vi "Sensors - Create New Calibration Table from File.vi"(0 "Calibration Data File":path, 5 "Conversion Type":T1, 9 "New Calibration Data File":path, 11 "Write table to file":bool) -> (4 "Output Table":dbl[][](array[numeric]) format="%.4f")   [LabVIEW 2011]
uses:
  Sensors - Controls/Sensors - Conversion Type.ctl
  <vilib>/Analysis/NI_AALPro.lvlib
panel:
  out "Table - Original & Created Data":cluster{dbl[], dbl[]}[](graph)
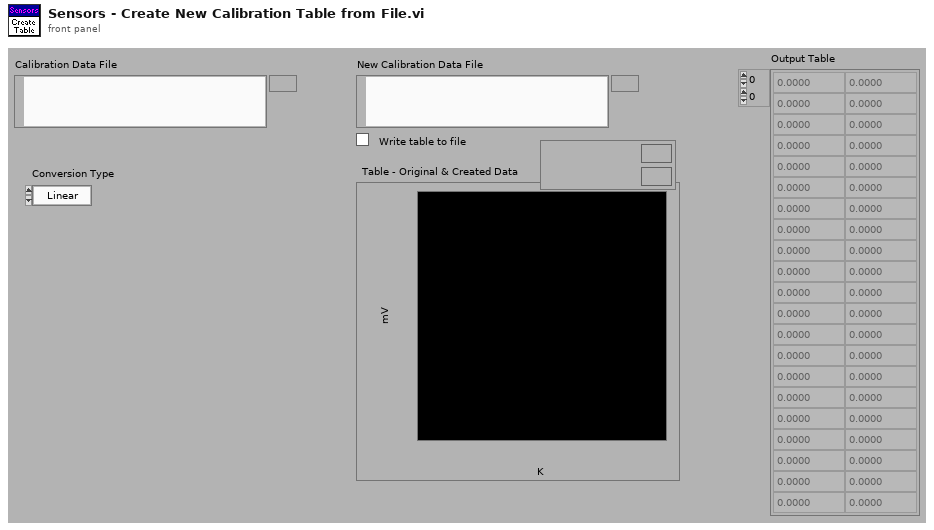
[diagram p1: front panel]
types:
  T1 = typedef "Sensors - Conversion Type.ctl" = enum16{"Linear", "Spline"}
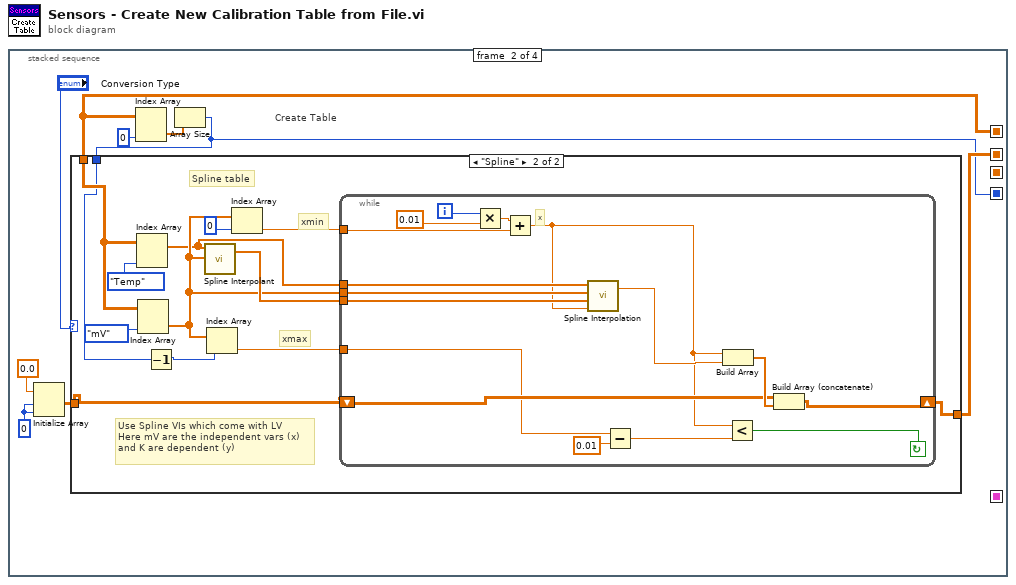
[diagram p0: block diagram]
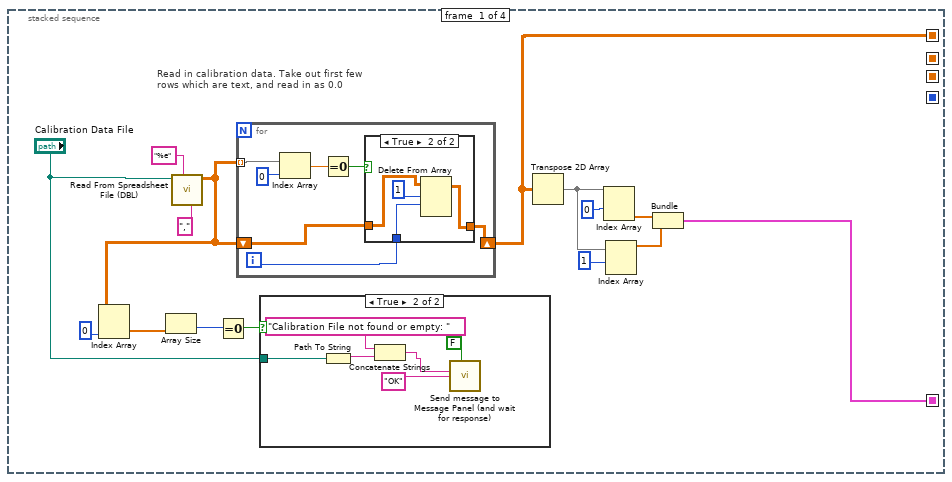
[diagram p2: hidden frame]
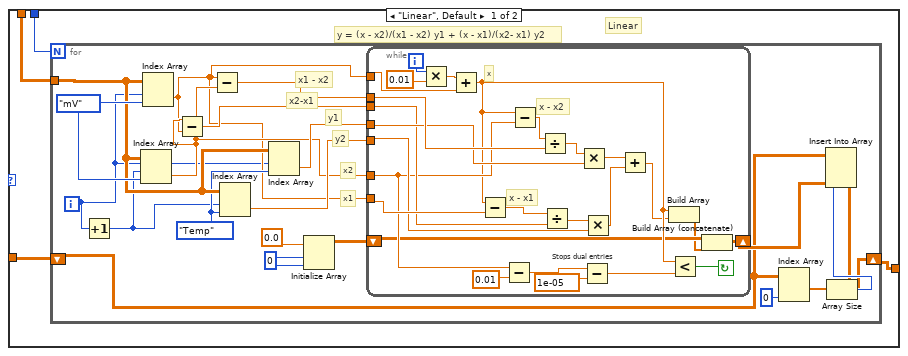
[diagram p5: hidden frame]
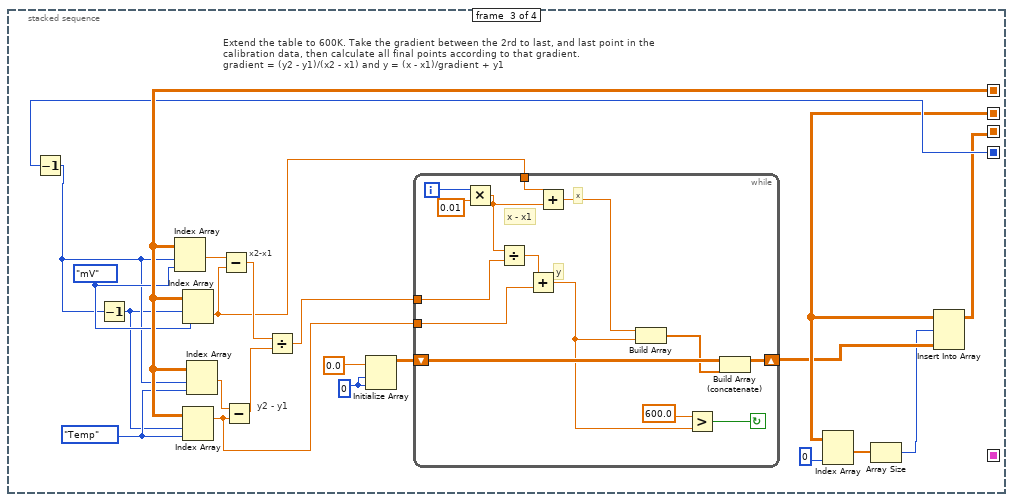
[diagram p6: hidden frame]
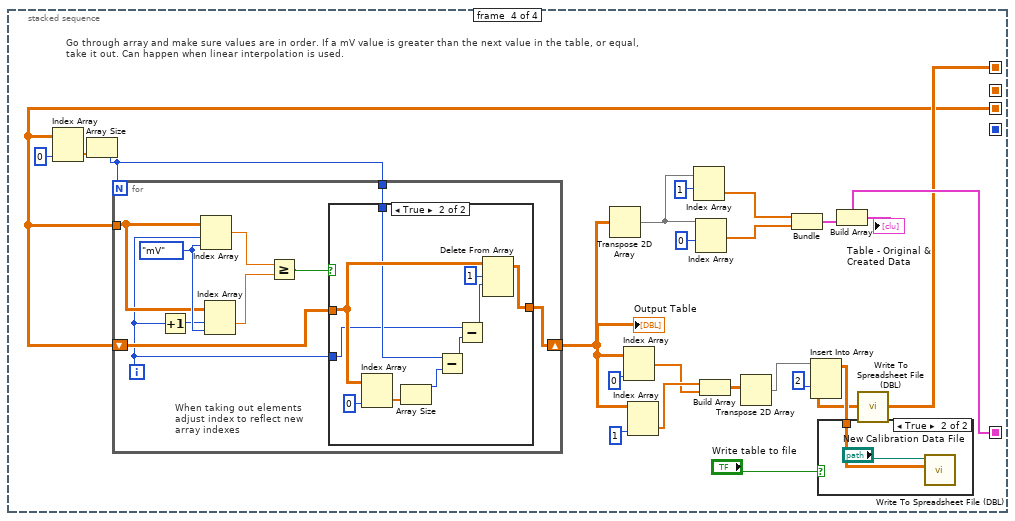
[diagram p7: hidden frame]
diagram:
  n1 = stacked-sequence {
    seq-local: [w8 _ _ _] -> [_ w37 w143 w163]
    seq-local: [_ w36 _ _] -> [_ _ w141 _]
    seq-local: [w1 _ _ _] -> [_ _ _ w172]
    seq-local: [_ w35 _ _] -> [_ _ w142 _]
    seq-local: [_ _ w140 _] -> [_ _ _ w161]
    frame #0 {
      # "Read in calibration data. Take out first few\nrows which are text, and read in as 0.0"
      n2 = call <vilib>:"Read From Spreadsheet File (DBL).vi"("delimiter (\\t)"=",", "format (%.3f)"="%e", "file path (dialog if empty)"="Calibration Data File") -> ("all rows"=w6:dbl[][])  [unwired: 4 in, 4 out]
      n3 = Index Array(array=w6, index (col)=0) -> (element=w4:dbl[])  [unwired: 1 in]
      n4 = Array Size(array=w4) -> (size(s)=w7:i32)
      n5 = Equal To 0?(x=w7) -> (x = 0?=w3:bool)
      n6 = for {
        tunnel: w6 -> [w28] mode=indexing
        shift-right: [w23] -> w8
        shift-left: w6 -> [w24]
        i -> [w22]
        n7 = Index Array(array=w28, index=0) -> (element=w26:dbl)
        n8 = Equal To 0?(x=w26) -> (x = 0?=w25:bool)
        n9 = case shown="True" w25 {
          tunnel: w24 -> [w29 w32]
          tunnel: [w29 w30] -> w23
          tunnel: w22 -> [_ w31]
          frame False {
          }
          frame True {
            n10 = Delete From Array(array=w32, length=1, index (row)=w31) -> (array with subset deleted=w30:dbl[][])  [unwired: 1 in, 1 out]
          }
        }
      }
      n11 = case shown="True" w3 {
        tunnel: "Calibration Data File" -> [_ w19]
        frame False {
        }
        frame True {
          n12 = Path To String(path=w19) -> (string=w20:string)
          n13 = Concatenate Strings("Calibration File not found or empty: ", w20) -> (w18:string)
          n14 = call "Send message to Message Panel (and wait for response).vi"("Prompt"=w18, "Wait for response?"=FALSE, "Yes text"="OK") -> ()  [unwired: 2 in, 1 out]
        }
      }
      n15 = Transpose 2D Array(2D array=w8) -> (transposed array=w13:dbl[][])
      n16 = Index Array(array=w13, index (row)=0) -> (element=w15:dbl[])  [unwired: 1 in]
      n17 = Index Array(array=w13, index (row)=1) -> (element=w14:dbl[])  [unwired: 1 in]
      n18 = Bundle(w15, w14) -> (w1:cluster{dbl[], dbl[]})  [unwired: 1 in]
    }
    frame #1 {
      w40 = 0
      # "Create Table"
      n19 = Initialize Array(0.0, w40, w40) -> (w42:dbl[][])
      n20 = Index Array(array=w37, index (col)=0) -> (element=w39:dbl[])  [unwired: 1 in]
      n21 = Array Size(array=w39) -> (size(s)=w35:i32)
      n22 = case shown="\"Spline\"" "Conversion Type" {
        tunnel: w42 -> [w46 w105]
        tunnel: w37 -> [w45 w102]
        tunnel: [w44 w93] -> w36
        tunnel: w35 -> [w43 w100]
        frame "Linear", Default {
          # "Linear"
          # "y = (x - x2)/(x1 - x2) y1 + (x - x1)/(x2- x1) y2"
          n23 = for {
            N: w43 -> [_]
            tunnel: w45 -> [w65]
            shift-right: [w50] -> w44
            shift-left: w46 -> [w54]
            i -> [w56]
            w47 = 0
            w64 = enum16{"Temp", "mV"}."Temp"
            w66 = enum16{"Temp", "mV"}."mV"
            # "x1"
            # "x2"
            # "y1"
            # "y2"
            # "x1 - x2"
            # "x2-x1"
            n24 = Increment(x=w56) -> (x+1=w57:i32)
            n25 = Index Array(array=w65, index (row)=w57, index (col)=w66) -> (element=w59:dbl)
            n26 = Index Array(array=w65, index (row)=w56, index (col)=w66) -> (element=w58:dbl)
            n27 = Subtract(x=w59, y=w58) -> (x-y=w62:dbl)
            n28 = Subtract(x=w58, y=w59) -> (x-y=w63:dbl)
            n29 = Index Array(array=w65, index (row)=w57, index (col)=w64) -> (element=w60:dbl)
            n30 = Index Array(array=w65, index (row)=w56, index (col)=w64) -> (element=w61:dbl)
            n31 = Initialize Array(0.0, w47, w47) -> (w48:dbl[][])
            n32 = while {
              tunnel: w63 -> [w91]
              tunnel: w62 -> [w85]
              tunnel: w61 -> [w89]
              tunnel: w60 -> [w83]
              tunnel: w59 -> [w77]
              tunnel: w58 -> [w87]
              tunnel: w58 -> [w78]
              shift-right: [w69] -> w55
              shift-left: w48 -> [w71]
              i -> [w80]
              stop <- w72 continue-if-true
              # "Stops dual entries"
              # "x - x1"
              # "x"
              # "x - x2"
              n33 = Multiply(x=w80, y=0.01) -> (x*y=w81:dbl)
              n34 = Add(x=w81, y=w78) -> (x+y=w74:dbl)
              n35 = Subtract(x=w74, y=w87) -> (x-y=w86:dbl)
              n36 = Subtract(x=w77, y=0.01) -> (x-y=w75:dbl)
              n37 = Subtract(x=w74, y=w77) -> (x-y=w92:dbl)
              n38 = Divide(x=w92, y=w91) -> (x/y=w90:dbl)
              n39 = Divide(x=w86, y=w85) -> (x/y=w84:dbl)
              n40 = Multiply(x=w90, y=w89) -> (x*y=w88:dbl)
              n41 = Subtract(x=w75, y=1e-05) -> (x-y=w68:dbl)
              n42 = Multiply(x=w84, y=w83) -> (x*y=w82:dbl)
              n43 = Add(x=w88, y=w82) -> (x+y=w73:dbl)
              n44 = Build Array(w74, w73) -> (w70:dbl[])
              n45 = Less?(x=w74, y=w68) -> (x < y?=w72:bool)
              n46 = Build Array (concatenate)(w71, w70) -> (w69:dbl[][])
            }
            n47 = Index Array(array=w54, index (col)=0) -> (element=w52:dbl[])  [unwired: 1 in]
            n48 = Array Size(array=w52) -> (size(s)=w51:i32)
            n49 = Insert Into Array(array=w54, index (row)=w51, new element=w55) -> (w50:dbl[][])  [unwired: 1 in]
          }
        }
        frame "Spline" {
          # "Spline table"
          # "Use Spline VIs which come with LV\nHere mV are the independent vars (x)\nand K are dependent (y)"
          # "xmin"
          # "xmax"
          n50 = Index Array(array=w102, index (col)=enum16{"Temp", "mV"}."Temp") -> (element=w94:dbl[])  [unwired: 1 in]
          n51 = Index Array(array=w102, index (col)=enum16{"Temp", "mV"}."mV") -> (element=w95:dbl[])  [unwired: 1 in]
          n52 = Decrement(x=w100) -> (x-1=w101:i32)
          n53 = call <vilib>:"Spline Interpolant.vi"("X"=w95, "Y"=w94) -> ("Interpolant"=w98:dbl[])  [unwired: 2 in, 1 out]
          n54 = Index Array(array=w95, index=w101) -> (element=w99:dbl)
          n55 = Index Array(array=w95, index=0) -> (element=w96:dbl)
          n56 = while {
            shift-right: [w116] -> w93
            shift-left: w105 -> [w115]
            tunnel: w98 -> [w113]
            tunnel: w99 -> [w107]
            tunnel: w96 -> [w109]
            tunnel: w95 -> [w111]
            tunnel: w94 -> [w110]
            i -> [w114]
            stop <- w106 continue-if-true
            # "x"
            n57 = Multiply(x=w114, y=0.01) -> (x*y=w121:dbl)
            n58 = Add(x=w121, y=w109) -> (x+y=w108:dbl)
            n59 = call <vilib>:"Spline Interpolation.vi"("x value"=w108, "Interpolant"=w113, "X"=w111, "Y"=w110) -> ("interpolation value"=w112:dbl)  [unwired: 1 out]
            n60 = Subtract(x=w107, y=0.01) -> (x-y=w118:dbl)
            n61 = Build Array(w108, w112) -> (w117:dbl[])
            n62 = Less?(x=w108, y=w118) -> (x < y?=w106:bool)
            n63 = Build Array (concatenate)(w115, w117) -> (w116:dbl[][])
          }
        }
      }
    }
    frame #2 {
      w131 = 0
      w138 = enum16{"Temp", "mV"}."Temp"
      w139 = enum16{"Temp", "mV"}."mV"
      # "y2 - y1"
      # "x2-x1"
      # "Extend the table to 600K. Take the gradient between the 2rd to last, and last point in the \ncalibration data, then calculate all final points according to that gradient. \ngradient = (y2 - y1)/(x2 - x1) and y = (x - x1)/gradient + y1"
      n64 = Decrement(x=w142) -> (x-1=w129:i32)
      n65 = Decrement(x=w129) -> (x-1=w128:i32)
      n66 = Index Array(array=w143, index (row)=w129, index (col)=w139) -> (element=w130:dbl)
      n67 = Index Array(array=w143, index (row)=w128, index (col)=w139) -> (element=w124:dbl)
      n68 = Index Array(array=w143, index (row)=w128, index (col)=w138) -> (element=w122:dbl)
      n69 = Index Array(array=w143, index (row)=w129, index (col)=w138) -> (element=w127:dbl)
      n70 = Subtract(x=w130, y=w124) -> (x-y=w125:dbl)
      n71 = Subtract(x=w127, y=w122) -> (x-y=w126:dbl)
      n72 = Divide(x=w125, y=w126) -> (x/y=w123:dbl)
      n73 = Initialize Array(0.0, w131, w131) -> (w132:dbl[][])
      n74 = while {
        shift-right: [w152] -> w137
        shift-left: w132 -> [w154]
        tunnel: w124 -> [w147]
        tunnel: w123 -> [w146]
        tunnel: w122 -> [w150]
        i -> [w157]
        stop <- w155 continue-if-true
        # "y"
        # "x - x1"
        # "x"
        n75 = Multiply(x=w157, y=0.01) -> (x*y=w144:dbl)
        n76 = Divide(x=w144, y=w146) -> (x/y=w145:dbl)
        n77 = Add(x=w145, y=w150) -> (x+y=w149:dbl)
        n78 = Add(x=w147, y=w144) -> (x+y=w148:dbl)
        n79 = Build Array(w148, w149) -> (w153:dbl[])
        n80 = Greater?(x=600.0, y=w149) -> (0:w155:bool)
        n81 = Build Array (concatenate)(w154, w153) -> (w152:dbl[][])
      }
      n82 = Index Array(array=w141, index (col)=0) -> (element=w135:dbl[])  [unwired: 1 in]
      n83 = Array Size(array=w135) -> (size(s)=w134:i32)
      n84 = Insert Into Array(array=w141, index (row)=w134, new element=w137) -> (w140:dbl[][])  [unwired: 1 in]
    }
    frame #3 {
      # "Go through array and make sure values are in order. If a mV value is greater than the next value in the table, or equal, \ntake it out. Can happen when linear interpolation is used."
      n85 = Index Array(array=w161, index (col)=0) -> (element=w174:dbl[])  [unwired: 1 in]
      n86 = Array Size(array=w174) -> (size(s)=w180:i32)
      n87 = for {
        N: w180 -> [_]
        tunnel: w161 -> [w187]
        shift-right: [w185] -> w158
        shift-left: w161 -> [w186]
        tunnel: w180 -> [w183]
        i -> [w184]
        w192 = enum16{"Temp", "mV"}."mV"
        # "When taking out elements\nadjust index to reflect new \narray indexes"
        n88 = Increment(x=w184) -> (x+1=w191:i32)
        n89 = Index Array(array=w187, index (row)=w184, index (col)=w192) -> (element=w190:dbl)
        n90 = Index Array(array=w187, index (row)=w191, index (col)=w192) -> (element=w189:dbl)
        n91 = Greater Or Equal?(x=w190, y=w189) -> (x >= y?=w188:bool)
        n92 = case shown="True" w188 {
          tunnel: w186 -> [w193 w199]
          tunnel: [w193 w203] -> w185
          tunnel: w184 -> [_ w196]
          tunnel: w183 -> [_ w198]
          frame False {
          }
          frame True {
            n93 = Index Array(array=w199, index (col)=0) -> (element=w200:dbl[])  [unwired: 1 in]
            n94 = Array Size(array=w200) -> (size(s)=w197:i32)
            n95 = Subtract(x=w198, y=w197) -> (x-y=w195:i32)
            n96 = Subtract(x=w196, y=w195) -> (x-y=w194:i32)
            n97 = Delete From Array(array=w199, length=1, index (row)=w194) -> (array with subset deleted=w203:dbl[][])  [unwired: 1 in, 1 out]
          }
        }
      }
      "Output Table" <- w158
      n98 = Transpose 2D Array(2D array=w158) -> (transposed array=w176:dbl[][])
      n99 = Index Array(array=w158, index (col)=0) -> (element=w165:dbl[])  [unwired: 1 in]
      n100 = Index Array(array=w158, index (col)=1) -> (element=w166:dbl[])  [unwired: 1 in]
      n101 = Index Array(array=w176, index (row)=1) -> (element=w177:dbl[])  [unwired: 1 in]
      n102 = Index Array(array=w176, index (row)=0) -> (element=w178:dbl[])  [unwired: 1 in]
      n103 = Build Array(w166, w165) -> (w164:dbl[][])
      n104 = Transpose 2D Array(2D array=w164) -> (transposed array=w162:dbl[][])
      n105 = Bundle(w177, w178) -> (w171:cluster{dbl[], dbl[]})  [unwired: 1 in]
      n106 = Insert Into Array(array=w162, index (col)=2, new element=w163) -> (w170:dbl[][])  [unwired: 1 in]
      n107 = case shown="True" "Write table to file" {
        tunnel: w170 -> [_ w182]
        frame False {
        }
        frame True {
          n108 = call <vilib>:"Write To Spreadsheet File (DBL).vi"("2D data"=w182) -> ()  [unwired: 7 in, 1 out]
          n109 = call <vilib>:"Write To Spreadsheet File (DBL).vi"("2D data"=w182, "file path (dialog if empty)"="New Calibration Data File") -> ()  [unwired: 6 in, 1 out]
        }
      }
      n110 = Build Array(w172, w171) -> (→"Table - Original & Created Data":cluster{dbl[], dbl[]}[])
    }
  }
